vi "Init VI.vi"(8 "error in (no error)":errorcluster, 11 "Rigol DG822 Pulse in":refnum<class "Rigol DG822 Pulse.lvclass">) -> (0 "error out":errorcluster, 3 "Rigol DG822 Pulse out":refnum<class "Rigol DG822 Pulse.lvclass">)   [LabVIEW 2021, in "Rigol DG822 UI.lvlib" / "Rigol DG822 Pulse.lvlib" / "Rigol DG822 Pulse.lvclass"]
uses:
  Rigol DG822 Pulse.lvclass
  D:/LabVIEW/General/Files/lvlibp/Actor Framework.lvlibp/1abvi3w/vi.lib/ActorFramework/Actor/Actor.lvclass
  Rigol DG822 Pulse.lvclass/Rigol DG822 Pulse.ctl
  General/Files/lvlibp/Actors.lvlibp/Actors/Actors/Actors.lvclass
  General/Files/lvlibp/Actor Framework.lvlibp/1abvi3w/vi.lib/ActorFramework/Actor/Actor.lvclass
  D:/LabVIEW/General/Files/lvlibp/Actors.lvlibp/Actors/Actors/Actors.lvclass
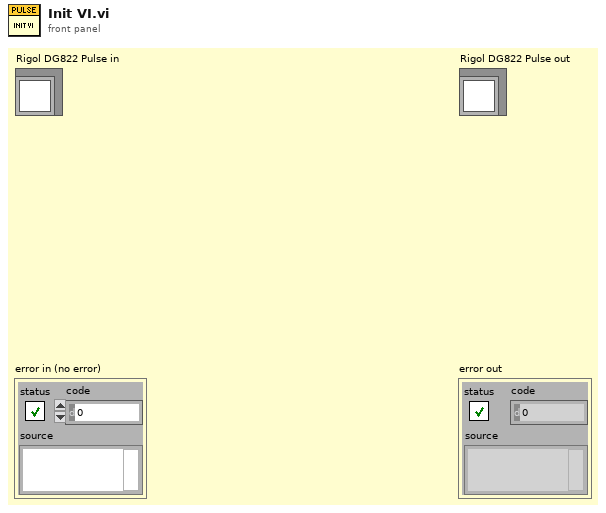
[diagram p1: front panel]
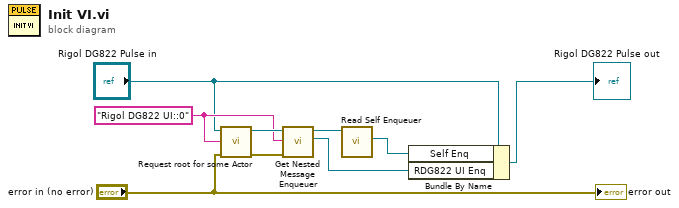
[diagram p0: block diagram]
diagram:
  w6 = "Rigol DG822 UI::0" ("Actor Name")
  n1 = call "Request root for some Actor.vi"("error in (no error)"="error in (no error)", "Actor Name"=w6, "Actors in"="Rigol DG822 Pulse in") -> ("error out"=w7:errorcluster, "Actors out"=w8:refnum<class "Rigol DG822 Pulse.lvclass">)  [unwired: 7 in]
  n2 = call "Get Nested Message Enqueuer.vi"("Actor name ()"=w6, "error in (no error)"=w7, "Actors in"=w8) -> ("Message Enqueuer"=w5:refnum<class "Message Enqueuer.lvclass">, "Actors out"=w9:refnum<class "Rigol DG822 Pulse.lvclass">)  [unwired: 4 in, 3 out]
  n3 = call "Read Self Enqueuer.vi"("Actor"=w9) -> ("Self Enqueuer"=w4:refnum<class "Message Enqueuer.lvclass">)  [unwired: 10 in]
  n4 = Bundle By Name(cluster="Rigol DG822 Pulse in", "Self Enq"=w4, "RDG822 UI Enq"=w5) -> (→"Rigol DG822 Pulse out":refnum<class "Rigol DG822 Pulse.lvclass">)
  "error out" <- "error in (no error)"
